vi "ControlMotorSetIo.vi"(3 "状态":bool, 5 "动作IO":enum16{"俯仰轴归0", "旋转轴归0", "空"}(ring)) -> (1 "handle out":u32)   [LabVIEW 2018]
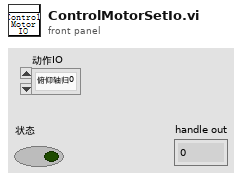
[diagram p1: front panel]
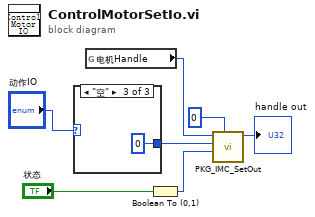
[diagram p0: block diagram]
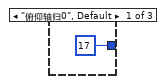
[diagram p2: hidden frame]
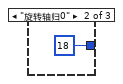
[diagram p3: hidden frame]
diagram:
  n1 = case shown="\"空\"" "动作IO" {
    tunnel: [17 18 0] -> w2
    frame "俯仰轴归0", Default {
    }
    frame "旋转轴归0" {
    }
    frame "空" {
    }
  }
  n2 = global read "参数.vi" "电机Handle"() -> (w7:u32)
  n3 = Boolean To (0,1)(Boolean="状态") -> (0, 1=w4:i16)
  n4 = call "PKG_IMC_SetOut.vi"("fifo"=0, "data"=w4, "outPort"=w2, "handle"=w7) -> ("handle out"=→"handle out":u32)  [unwired: 6 in, 1 out]
